vi "Serial Data clean.vi"(3 "string":string) -> (1 "Stripped of Xon Xoff":string)   [LabVIEW 2020]
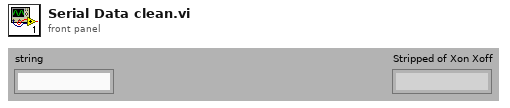
[diagram p1: front panel]
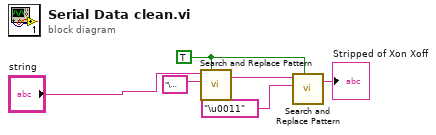
[diagram p0: block diagram]
diagram:
  w1 = TRUE ("replace all? (F)")
  n1 = call "Search and Replace Pattern.vi"("string"="string", "regular expression (\"\")"="\u0013" ("regular expression (\"\")"), "replace all? (F)"=w1) -> ("result string"=w5:string)  [unwired: 2 in, 1 out]
  n2 = call "Search and Replace Pattern.vi"("string"=w5, "regular expression (\"\")"="\u0011" ("regular expression (\"\")"), "replace all? (F)"=w1) -> ("result string"=→"Stripped of Xon Xoff":string)  [unwired: 2 in, 1 out]
